vi "Event Logger.vi"(10 "Panel":refnum<class "Panel.lvclass">, 11 "Command":refnum<user-event>) -> ()   [LabVIEW 2017, in "1. Basic Panels.lvlib"]
doc: "This is a basic panel. \n\nIt doesn't know what type of panel it is until runtime, this means that whoever launches this VI can define what type of panel it will be.\n----\nCopyright: MGI 2016\nAuthor: Derek Trepanier"
uses:
  1. Basic Panels.lvlib
  panel-manager/Source/Panel/Panel.lvclass
  panel-manager/Source/Panel Helper/Panel Helper.lvclass
panel:
  out "Event Log":string
  out "Top Level Panel":string
  in  "Show":bool
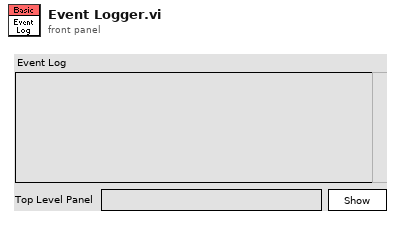
[diagram p1: front panel]
types:
  T1 = cluster{"Panel":refnum<event-registration>, "Event Registration Refnum":refnum<event-registration>}
  T2 = typedef "Panel.lvlib/Panel Helper.lvclass/Events.ctl" = enum16{"Initialized", "Shown", "Hidden", "Closed"}
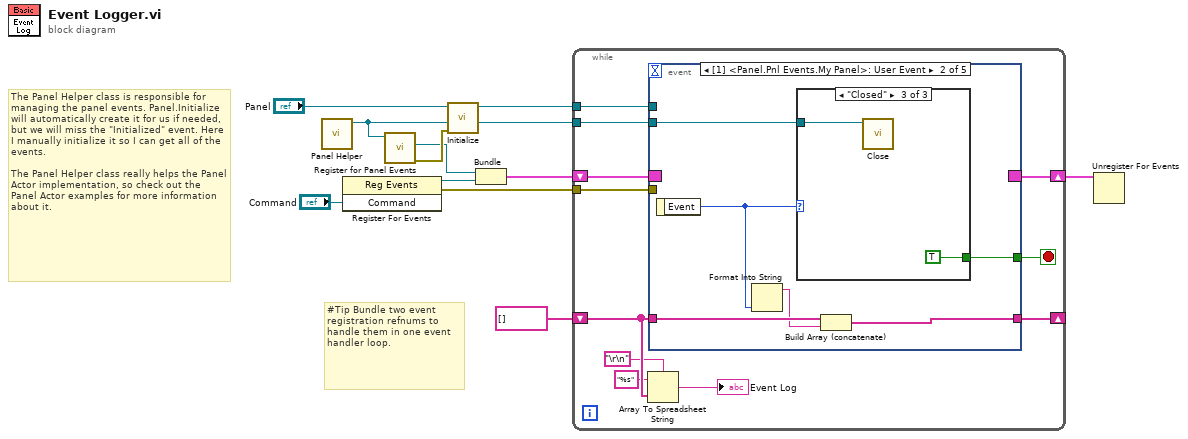
[diagram p0: block diagram]
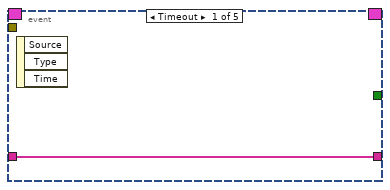
[diagram p2: hidden frame]
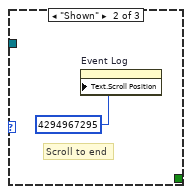
[diagram p4: hidden frame]
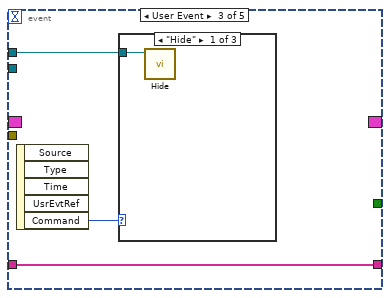
[diagram p5: hidden frame]
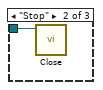
[diagram p6: hidden frame]
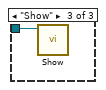
[diagram p7: hidden frame]
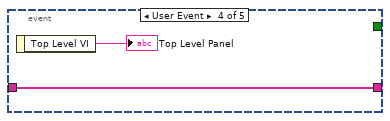
[diagram p8: hidden frame]
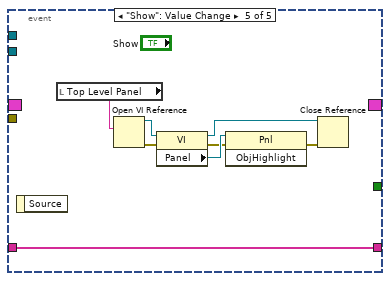
[diagram p9: hidden frame]
diagram:
  # "The Panel Helper class is responsible for managing the panel events. Panel.Initialize will automatically create it for us if needed, but we will miss the \"Initialized\" event. Here I manually initialize it so I can get all of the events.\n\nThe Panel Helper class really helps the Panel Actor implementation, so check out the Panel Actor examples for more information about it."
  # "#Tip Bundle two event registration refnums to handle them in one event handler loop."
  n1 = call "Panel Helper.vi"() -> ("Panel Helper out"=w7:refnum<class "Panel Helper.lvclass">)  [unwired: 9 in, 2 out]
  n2 = register-events("Command") -> (reference out=w11:refnum<event-registration>, error out=w8:errorcluster)  [unwired: 2 in]
  n3 = call "Register for Panel Events.vi"("Panel Helper in"=w7) -> ("error out"=w6:errorcluster, "Panel"=w1:refnum<event-registration>)  [unwired: 9 in]
  n4 = call "Initialize.vi"("error in (no error)"=w6, "My Helper in"=w7, "Panel In"="Panel") -> ("My Helper out"=w4:refnum<class "Panel Helper.lvclass">, "Panel Out"=w10:refnum<class "Panel.lvclass">)  [unwired: 6 in, 1 out]
  n5 = Bundle("Panel"=w1, "Event Registration Refnum"=w11) -> (w5:T1)  [unwired: 1 in]
  n6 = while {
    tunnel: w8 -> [w20]
    shift-right: [w21] -> w9
    shift-left: w5 -> [w23]
    tunnel: w4 -> [w18]
    tunnel: w10 -> [w22]
    shift-right: [w17] -> _
    shift-left: string[] [] -> [w16]
    stop <- w19 stop-if-true
    n7 = Array To Spreadsheet String(delimiter (Tab)="\r\n", array=w16, 3:"%s" ("format string")) -> (spreadsheet string=→"Event Log":string)
    n8 = event shown="[1] <Panel.Pnl Events.My Panel>: User Event" {
      selector: w23 -> [_ _ _ _ _]
      dyn-events: [_ _ _ _ _] -> w21
      timeout: _ -> [_ _ _ _ _]
      tunnel: w22 -> [_ _ w36 _ _]
      tunnel: w20 -> [_ _ _ _ _]
      tunnel: [_ w29 _ _ _] -> w19
      tunnel: w18 -> [_ w30 _ _ _]
      tunnel: w16 -> [w24 w28 w35 w41 w49]
      tunnel: [w24 w27 w35 w41 w49] -> w17
      event Timeout {
        n9 = event-data() -> ()  [unwired: 1 in, 3 out]
      }
      event User Event {
        n10 = event-data() -> ("Event"=w26:T2)  [unwired: 1 in]
        n11 = Format Into String(w26) -> (resulting string=w25:string)  [unwired: 3 in, 1 out]
        n12 = case shown="\"Closed\"" w26 {
          tunnel: w30 -> [_ _ w33]
          tunnel: [_ _ TRUE] -> w29
          frame Default {
          }
          frame "Shown" {
            # "Scroll to end"
            n13 = property on="Event Log" class="Str"("Text.Scroll Position"=u32 4294967295) -> ()  [unwired: 2 in, 2 out]
          }
          frame "Closed" {
            n14 = call "Close.vi"("Controller in"=w33) -> ()  [unwired: 10 in, 1 out]
          }
        }
        n15 = Build Array (concatenate)(w28, w25) -> (w27:string[])
      }
      event User Event {
        n16 = event-data() -> ("Command"=w34:enum16{"Show", "Hide", "Stop"})  [unwired: 1 in, 4 out]
        n17 = case shown="\"Hide\"" w34 {
          tunnel: w36 -> [w37 w38 w39]
          frame "Hide" {
            n18 = call "Hide.vi"("Panel In"=w37) -> ()  [unwired: 10 in, 1 out]
          }
          frame "Stop" {
            n19 = call-dynamic "Close.vi"("Panel In"=w38) -> ()  [unwired: 10 in, 1 out]
          }
          frame "Show" {
            n20 = call "Show.vi"("Panel in"=w39) -> ()  [unwired: 10 in, 1 out]
          }
        }
      }
      event User Event {
        n21 = event-data() -> ("Top Level VI"=→"Top Level Panel":string)  [unwired: 1 in]
      }
      event "Show": Value Change {
        n22 = event-data() -> ()  [unwired: 1 in, 1 out]
        n23 = local read "Top Level Panel"() -> (w42:string)
        n24 = Open VI Reference(vi path=w42) -> (vi reference=w48:refnum<vi>, error out=w45:errorcluster)  [unwired: 5 in]
        n25 = property class="VI"(reference=w48, error in=w45) -> (reference out=w47:refnum<vi>, error out=w44:errorcluster, "Panel"=w46:refnum<vi>)
        n26 = invoke class="Pnl" method="ObjHighlight"(reference=w46, error in=w44) -> (error out=w43:errorcluster)  [unwired: 1 in, 2 out]
        n27 = Close Reference(reference=w47, error in (no error)=w43) -> ()  [unwired: 1 out]
      }
    }
  }
  n28 = Unregister For Events(event registration refnum=w9) -> ()  [unwired: 1 in, 1 out]
